vi "MC_TOOL_Edit Configs_MAIN.vi"() -> (0 "error out":errorcluster)   [LabVIEW 2009]
doc: "A Producer-Consumer two-loop state machine template. This template uses the LPD Command Queues to drive its execution.\n\nThere are several advantages such as:\n- convenient error state control\n- the ability to pass data between states/loops/VIs via a variant\n- command history which is extremely valuable in troubleshooting when an error occurs\n\n\nAuthor: Mike Schultz (mschultz11711@gmail.com)"
uses:
  SRV VIs/Support/SRV_Command-Data Queue Data Type.ctl
panel:
  in  "Edit Sensors Config":bool
  in  "Edit System Config":bool
  in  "Edit Motors Config":bool
  out "System Config":string
  out "Config Directory":path
  in  "About":bool
  in  "stop":bool
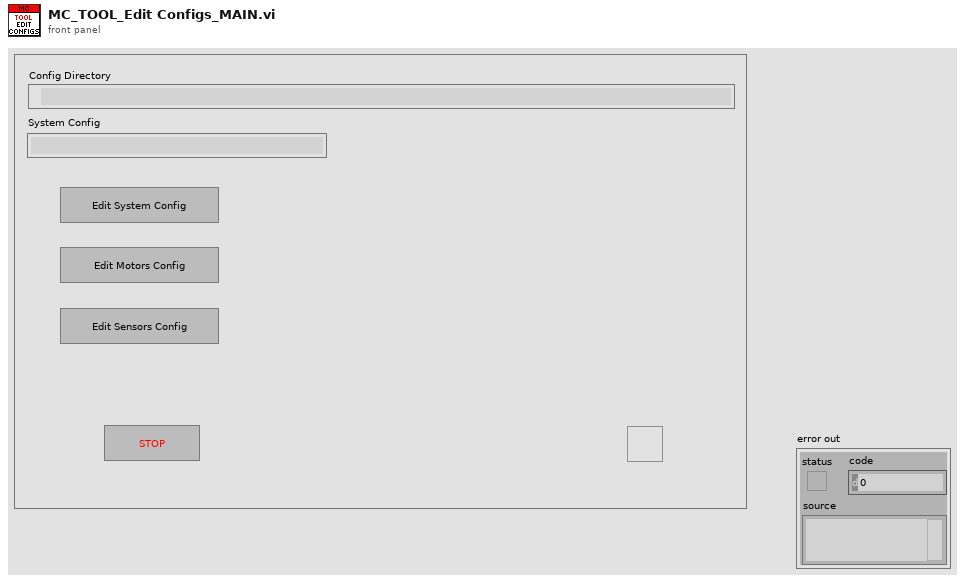
[diagram p1: front panel]
types:
  T1 = typedef "SRV_Command-Data Queue Data Type.ctl" = cluster{"Command":string, "Data":variant}
  T2 = cluster{"user event":refnum<user-event>, "Version":string, "Config Dir":path, "This VI ref":refnum<vi>, "System Config Name":string}
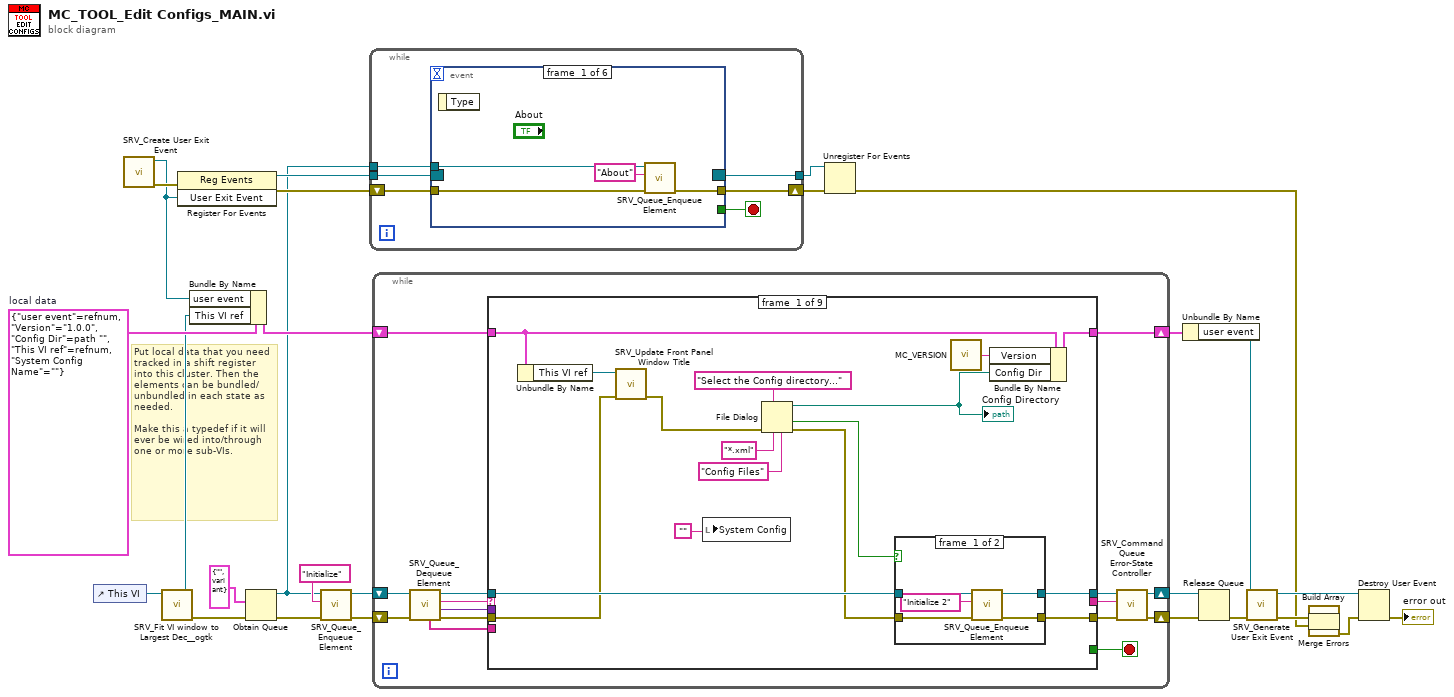
[diagram p0: block diagram]
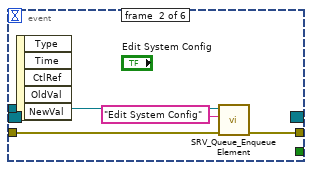
[diagram p2: hidden frame]
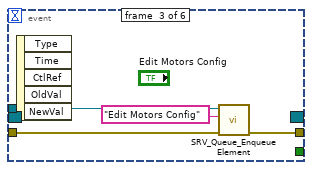
[diagram p3: hidden frame]
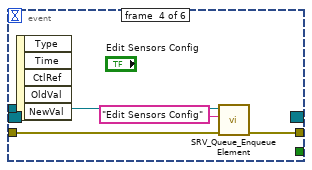
[diagram p4: hidden frame]
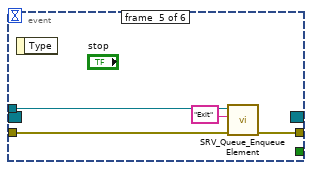
[diagram p5: hidden frame]
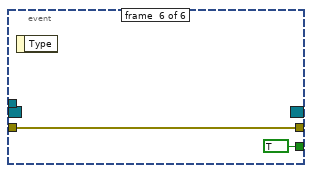
[diagram p6: hidden frame]
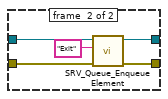
[diagram p7: hidden frame]
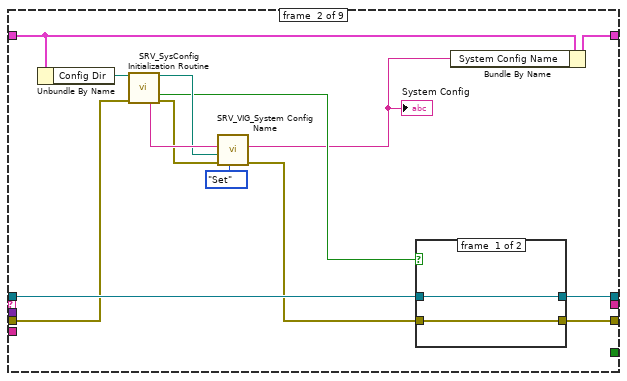
[diagram p8: hidden frame]
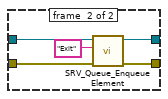
[diagram p9: hidden frame]
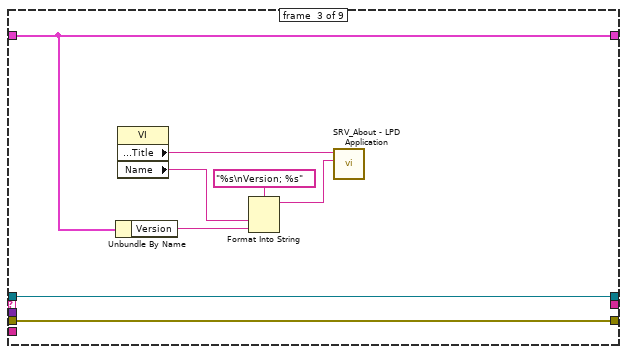
[diagram p10: hidden frame]
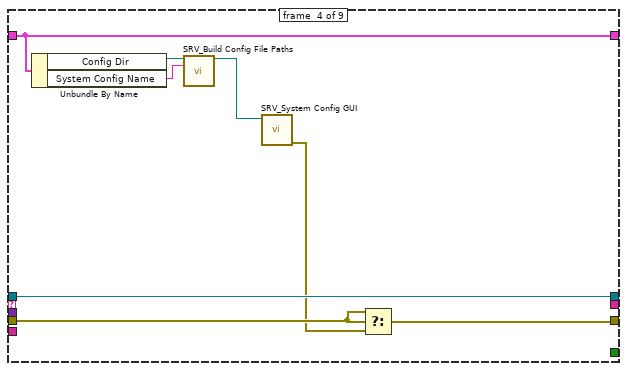
[diagram p11: hidden frame]
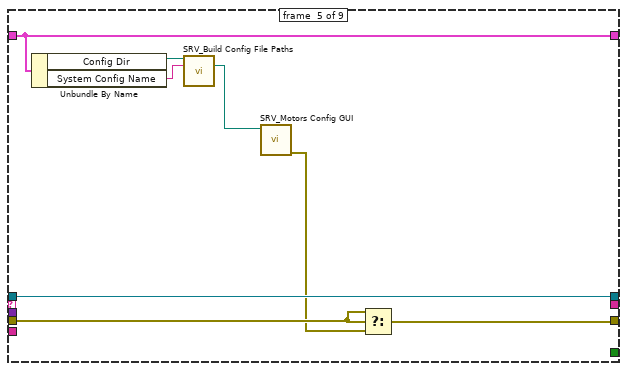
[diagram p12: hidden frame]
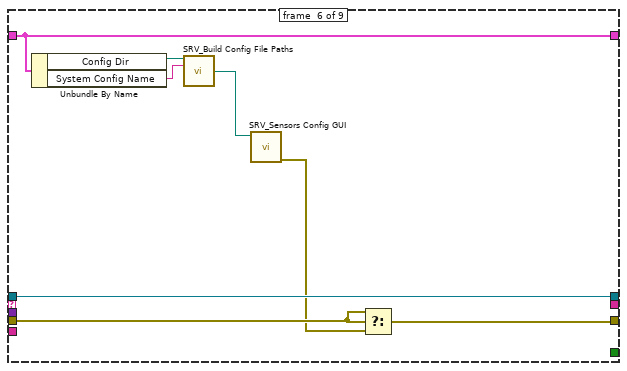
[diagram p13: hidden frame]
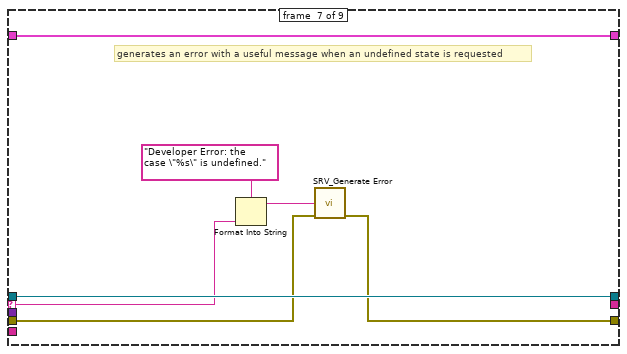
[diagram p14: hidden frame]
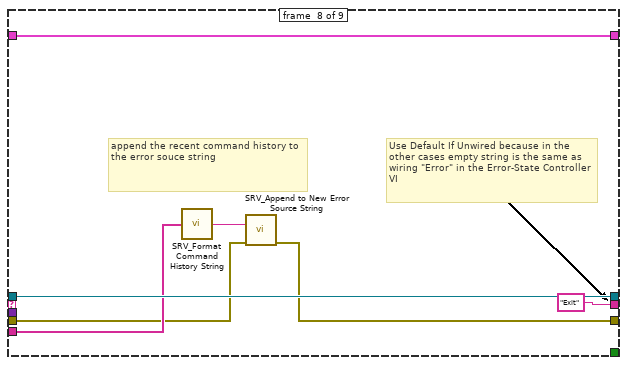
[diagram p15: hidden frame]
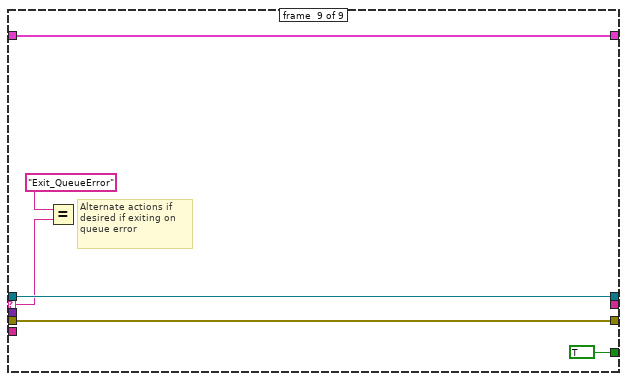
[diagram p16: hidden frame]
diagram:
  w21 = T2 {"user event"=refnum, "Version"="1.0.0", "Config Dir"=path "", "This VI ref"=refnum, "System Config Name"=""}  # local data
  # "Put local data that you need tracked in a shift register into this cluster. Then the elements can be bundled/unbundled in each state as needed.\n\nMake this a typedef if it will ever be wired into/through one or more sub-VIs."
  n1 = control-ref of="This VI"() -> (w2:refnum<vi>)
  n2 = call "SRV_Create User Exit Event.vi"() -> ("error out"=w12:errorcluster, "User Exit Event"=w11:refnum<user-event>)  [unwired: 10 in]
  n3 = call "SRV_Fit VI window to Largest Dec__ogtk.vi"("VI Ref (calling VI)"=w2) -> ("error out"=w5:errorcluster, "dup VI Ref"=w1:refnum<vi>)  [unwired: 5 in]
  n4 = register-events(error in=w12, w11) -> (reference out=w28:refnum<event-registration>, error out=w27:errorcluster)  [unwired: 1 in]
  n5 = Bundle By Name(cluster=w21, "user event"=w11, "This VI ref"=w1) -> (w20:T2)
  n6 = Obtain Queue(element data type=T1 {"Command"="", "Data"=variant} ("Queue Data Type"), error in (no error)=w5) -> (queue out=w7:refnum<queue>, error out=w8:errorcluster)  [unwired: 3 in, 1 out]
  n7 = call "SRV_Queue_Enqueue Element.vi"("error in (no error)"=w8, "Command"="Initialize", "Command-Data Queue"=w7) -> ("error out"=w3:errorcluster, "Command-Data Queue out"=w6:refnum<queue>)  [unwired: 6 in, 1 out]
  n8 = while {
    shift-right: [w29] -> w25
    shift-left: w27 -> [w34]
    tunnel: w7 -> [w33]
    tunnel: w28 -> [w32]
    tunnel: [w31] -> w26
    stop <- w30 stop-if-true
    n9 = event shown="[3] \"Edit Sensors Config\": Value Change" {
      selector: w32 -> [_ _ _ _ _ _]
      dyn-events: [_ _ _ _ _ _] -> w31
      timeout: _ -> [_ _ _ _ _ _]
      tunnel: w34 -> [w38 w40 w44 w48 w52 w56]
      tunnel: w33 -> [w35 w39 w43 w47 w51 _]
      tunnel: [_ _ _ _ _ TRUE] -> w30
      tunnel: [w37 w41 w45 w49 w53 w56] -> w29
      event #0 {
        n10 = event-data() -> ()  [unwired: 1 in, 1 out]
        n11 = call "SRV_Queue_Enqueue Element.vi"("error in (no error)"=w38, "Command"="About", "Command-Data Queue"=w35) -> ("error out"=w37:errorcluster)  [unwired: 6 in, 2 out]
      }
      event #1 {
        n12 = event-data() -> ()  [unwired: 1 in, 5 out]
        n13 = call "SRV_Queue_Enqueue Element.vi"("error in (no error)"=w40, "Command"="Edit System Config", "Command-Data Queue"=w39) -> ("error out"=w41:errorcluster)  [unwired: 6 in, 2 out]
      }
      event #2 {
        n14 = event-data() -> ()  [unwired: 1 in, 5 out]
        n15 = call "SRV_Queue_Enqueue Element.vi"("error in (no error)"=w44, "Command"="Edit Motors Config", "Command-Data Queue"=w43) -> ("error out"=w45:errorcluster)  [unwired: 6 in, 2 out]
      }
      event #3 {
        n16 = event-data() -> ()  [unwired: 1 in, 5 out]
        n17 = call "SRV_Queue_Enqueue Element.vi"("error in (no error)"=w48, "Command"="Edit Sensors Config", "Command-Data Queue"=w47) -> ("error out"=w49:errorcluster)  [unwired: 6 in, 2 out]
      }
      event #4 {
        n18 = event-data() -> ()  [unwired: 1 in, 1 out]
        n19 = call "SRV_Queue_Enqueue Element.vi"("error in (no error)"=w52, "Command"="Exit", "Command-Data Queue"=w51) -> ("error out"=w53:errorcluster)  [unwired: 6 in, 2 out]
      }
      event #5 {
        n20 = event-data() -> ()  [unwired: 1 in, 1 out]
      }
    }
  }
  n21 = while {
    shift-right: [w65] -> w24
    shift-left: w3 -> [w71]
    shift-right: [w63] -> w23
    shift-left: w6 -> [w69]
    shift-right: [w57] -> w19
    shift-left: w20 -> [w58]
    stop <- w59 stop-if-true
    n22 = call "SRV_Queue_Dequeue Element.vi"("error in (no error)"=w71, "Command-Data Queue"=w69) -> ("error out"=w70:errorcluster, "Data"=w62:variant, "Command"=w67:string, "Command-Data Queue out"=w68:refnum<queue>, "Command History"=w61:string[])  [unwired: 4 in, 1 out]
    n23 = case shown="\"About\"" w67 {
      selector: w67 -> [_ _ _ _ _ _ w155 _ w167]
      tunnel: w70 -> [w78 w105 w125 w129 w138 w146 w153 w159 w169]
      tunnel: [w85 w109 w125 w128 w137 w145 w152 w160 w169] -> w66
      tunnel: w68 -> [w87 w111 w126 w134 w142 w150 w157 w164 w170]
      tunnel: [w86 w110 w126 w134 w142 w150 w157 w164 w170] -> w64
      tunnel: w62 -> [_ _ _ _ _ _ _ _ _]
      tunnel: w61 -> [_ _ _ _ _ _ _ w163 _]
      tunnel: [_ _ _ _ _ _ _ "Exit" ("Error Command") _] -> w60
      tunnel: [_ _ _ _ _ _ _ _ TRUE] -> w59
      tunnel: w58 -> [w76 w108 w120 w133 w141 w149 w154 w161 w165]
      tunnel: [w75 w107 w120 w133 w141 w149 w154 w161 w165] -> w57
      frame #0 {
        n24 = Unbundle By Name(w76) -> ("This VI ref"=w79:refnum<vi>)
        n25 = call "SRV_Update Front Panel Window Title.vi"("error in (no error)"=w78, "VI ref"=w79) -> ("error out"=w77:errorcluster)  [unwired: 8 in, 1 out]
        n26 = local write "System Config"("") -> ()
        n27 = File Dialog(4:"Config Files" ("pattern label"), 6:"*.xml" ("pattern (all files)"), 7:"Select the Config directory..." ("prompt"), 8:w77) -> (0:w81:errorcluster, 1:w80:bool, 3:w73:path)  [unwired: 3 in, 1 out]
        "Config Directory" <- w73
        n28 = case shown="False" w80 {
          tunnel: w87 -> [w91 w97]
          tunnel: [w90 w96] -> w86
          tunnel: [w89 w95] -> w85
          tunnel: w81 -> [w88 w94]
          frame #0 {
            n29 = call "SRV_Queue_Enqueue Element.vi"("error in (no error)"=w88, "Command"="Initialize 2", "Command-Data Queue"=w91) -> ("error out"=w89:errorcluster, "Command-Data Queue out"=w90:refnum<queue>)  [unwired: 6 in, 1 out]
          }
          frame #1 {
            n30 = call "SRV_Queue_Enqueue Element.vi"("error in (no error)"=w94, "Command"="Exit", "Command-Data Queue"=w97) -> ("error out"=w95:errorcluster, "Command-Data Queue out"=w96:refnum<queue>)  [unwired: 6 in, 1 out]
          }
        }
        n31 = call "MC_VERSION.vi"() -> ("MC Version"=w74:string)
        n32 = Bundle By Name(cluster=w76, "Version"=w74, "Config Dir"=w73) -> (w75:T2)
      }
      frame #1 {
        n33 = Unbundle By Name(w108) -> ("Config Dir"=w106:path)
        n34 = call "SRV_SysConfig Initialization Routine.vi"("Config Dir"=w106, "error in (no error)"=w105) -> ("SystemConfig Filepath"=w102:path, "Cancelled?"=w101:bool, "Sys Config Name"=w103:string, "error out"=w100:errorcluster)  [unwired: 8 in, 2 out]
        n35 = call "SRV_VIG_System Config Name.vi"("Method (Get)"=enum16{"Get", "Set"}."Set", "error in (no error)"=w100, "SystemConfig Filepath"=w102, "System Config Name"=w103) -> ("error out"=w99:errorcluster, "System Config Name out"=w98:string)  [unwired: 5 in, 1 out]
        "System Config" <- w98
        n36 = case shown="False" w101 {
          tunnel: w111 -> [w113 w118]
          tunnel: [w113 w117] -> w110
          tunnel: [w112 w116] -> w109
          tunnel: w99 -> [w112 w115]
          frame #0 {
          }
          frame #1 {
            n37 = call "SRV_Queue_Enqueue Element.vi"("error in (no error)"=w115, "Command"="Exit", "Command-Data Queue"=w118) -> ("error out"=w116:errorcluster, "Command-Data Queue out"=w117:refnum<queue>)  [unwired: 6 in, 1 out]
          }
        }
        n38 = Bundle By Name(cluster=w108, "System Config Name"=w98) -> (w107:T2)
      }
      frame #2 {
        n39 = Unbundle By Name(w120) -> ("Version"=w119:string)
        n40 = property class="VI"() -> ("Front Panel.Title"=w124:string, "Name"=w121:string)  [unwired: 2 in, 2 out]
        n41 = Format Into String(format string="%s\nVersion; %s", w121, w119) -> (resulting string=w122:string)  [unwired: 2 in, 1 out]
        n42 = call "SRV_About - LPD Application.vi"("Version Info"=w122, "Application Name"=w124) -> ()  [unwired: 10 in]
      }
      frame #3 {
        n43 = Unbundle By Name(w133) -> ("Config Dir"=w132:path, "System Config Name"=w131:string)
        n44 = call "SRV_Build Config File Paths.vi"("Config Dir"=w132, "Sys Config Name"=w131) -> ("SystemConfig Filepath"=w130:path)  [unwired: 8 in, 5 out]
        n45 = call "SRV_System Config GUI.vi"("System Config File Path in"=w130) -> ("error out"=w127:errorcluster)  [unwired: 8 in, 2 out]
        n46 = Select(t=w129, s=w129, f=w127) -> (s? t:f=w128:errorcluster)
      }
      frame #4 {
        n47 = Unbundle By Name(w141) -> ("Config Dir"=w140:path, "System Config Name"=w139:string)
        n48 = call "SRV_Build Config File Paths.vi"("Config Dir"=w140, "Sys Config Name"=w139) -> ("MotorsConfig Filepath"=w136:path)  [unwired: 8 in, 5 out]
        n49 = call "SRV_Motors Config GUI.vi"("Motors Config File Path in"=w136) -> ("error out"=w135:errorcluster)  [unwired: 8 in, 2 out]
        n50 = Select(t=w138, s=w138, f=w135) -> (s? t:f=w137:errorcluster)
      }
      frame #5 {
        n51 = Unbundle By Name(w149) -> ("Config Dir"=w148:path, "System Config Name"=w147:string)
        n52 = call "SRV_Build Config File Paths.vi"("Config Dir"=w148, "Sys Config Name"=w147) -> ("SensorsConfig Filepath"=w144:path)  [unwired: 8 in, 5 out]
        n53 = call "SRV_Sensors Config GUI.vi"("Sensors Config File Path in"=w144) -> ("error out"=w143:errorcluster)  [unwired: 8 in, 2 out]
        n54 = Select(t=w146, s=w146, f=w143) -> (s? t:f=w145:errorcluster)
      }
      frame #6 {
        # "generates an error with a useful message when an undefined state is requested"
        n55 = Format Into String(format string="Developer Error: the case \"%s\" is undefined.", w155) -> (resulting string=w151:string)  [unwired: 2 in, 1 out]
        n56 = call "SRV_Generate Error.vi"("Message"=w151, "error in (no error)"=w153) -> ("error out"=w152:errorcluster)  [unwired: 13 in]
      }
      frame #7 {
        # "Use Default If Unwired because in the other cases empty string is the same as wiring \"Error\" in the Error-State Controller VI"
        # "append the recent command history to the error souce string"
        n57 = call "SRV_Format Command History String.vi"("Command History"=w163) -> ("Command History String"=w158:string)  [unwired: 14 in]
        n58 = call "SRV_Append to New Error Source String.vi"("Message String to append"=w158, "Error In (no error)"=w159) -> ("error out"=w160:errorcluster)  [unwired: 13 in]
      }
      frame #8 {
        # "Alternate actions if desired if exiting on queue error"
        n59 = Equal?(x="Exit_QueueError", y=w167) -> ()  [unwired: 1 out]
      }
    }
    n60 = call "SRV_Command Queue Error-State Controller.vi"("error in (no error)"=w66, "Error Command"=w60, "Command-Data Queue"=w64) -> ("error out"=w65:errorcluster, "Command-Data Queue out"=w63:refnum<queue>)  [unwired: 7 in]
  }
  n61 = Unregister For Events(event registration refnum=w26, error in=w25) -> (error out=w14:errorcluster)
  n62 = Unbundle By Name(w19) -> ("user event"=w18:refnum<user-event>)
  n63 = Release Queue(queue=w23, error in (no error)=w24) -> (error out=w17:errorcluster)  [unwired: 1 in, 2 out]
  n64 = call "SRV_Generate User Exit Event.vi"("error in (no error)"=w17, "User Exit Event"=w18) -> ("error out"=w15:errorcluster, "User Exit Event out"=w16:refnum<user-event>)  [unwired: 8 in]
  n65 = Build Array(w15, w14) -> (w10:errorcluster[])
  n66 = call <vilib>:"Merge Errors.vi"("error array in"=w10) -> ("error out"=w13:errorcluster)  [unwired: 6 in]
  n67 = Destroy User Event(user event=w16, error in=w13) -> (error out=→"error out":errorcluster)
